vi "Format Direction.vi"(7 "Xbox Controller (T)":bool=TRUE, 11 "Direction in":cluster{"X Axis":dbl, "Y Axis":dbl}) -> (3 "Formated Direction out":cluster{dbl, dbl})   [LabVIEW 2024, in "Utils.lvlib"]
doc: "MIT Licence\nCopyright (c) 2024 David Grollier"
uses:
  Utils.lvlib
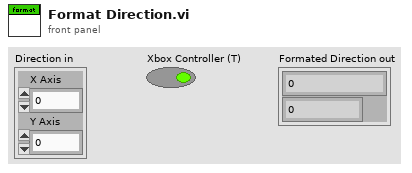
[diagram p1: front panel]
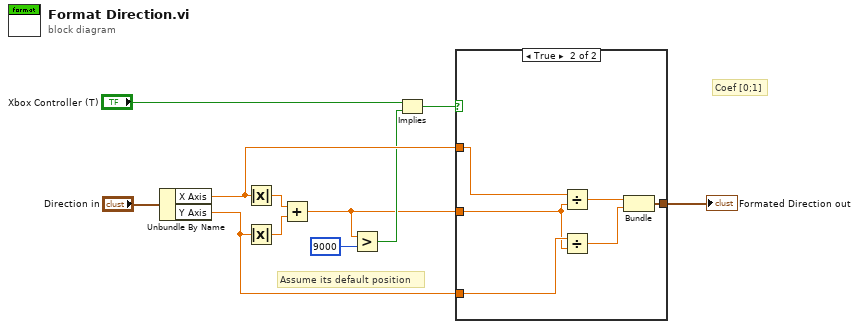
[diagram p0: block diagram]
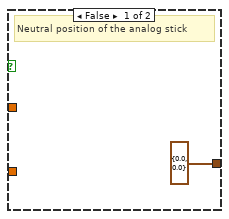
[diagram p2: hidden frame]
diagram:
  # "Coef [0;1]"
  # "Assume its default position"
  n1 = Unbundle By Name("Direction in") -> ("X Axis"=w10:dbl, "Y Axis"=w9:dbl)
  n2 = Absolute Value(x=w10) -> (abs(x)=w8:dbl)
  n3 = Absolute Value(x=w9) -> (abs(x)=w7:dbl)
  n4 = Add(x=w8, y=w7) -> (x+y=w3:dbl)
  n5 = Greater?(x=w3, y=9000) -> (0:w4:bool)
  n6 = Implies(1:w4, 2:"Xbox Controller (T)") -> (0:w2:bool)
  n7 = case shown="True" w2 {
    tunnel: [cluster{dbl, dbl} {0.0, 0.0} w18] -> w1
    tunnel: w10 -> [_ w15]
    tunnel: w9 -> [_ w14]
    tunnel: w3 -> [_ w13]
    frame False {
      # "Neutral position of the analog stick"
    }
    frame True {
      n8 = Divide(x=w15, y=w13) -> (x/y=w17:dbl)
      n9 = Divide(x=w14, y=w13) -> (x/y=w16:dbl)
      n10 = Bundle(w17, w16) -> (w18:cluster{dbl, dbl})  [unwired: 1 in]
    }
  }
  "Formated Direction out" <- w1
